vi "Get RGA Parameters.vi"(0 "Port Number":refnum<visa-resource-name>, 1 "error in (no error)":errorcluster) -> (2 "RGA Parameters":T1 {"Partial Pressure\nSensitivity Factor" format="%.3e"; "Steps/AMU" format="%.2f"; "Final Mass" format="%.2f"; "Initial Mass" format="%.2f"}, 4 "error out":errorcluster)   [LabVIEW 2025]
doc: "Author: Scott Hannahs <sth@magnet.fsu.edu>\n\nThis software is licensed for use under the “MIT License\"\nCopyright (c) 2025 Scott Hannahs, sth@sth@magnet.sthnet.net\n\nPermission is hereby granted, free of charge, to any person obtaining a copy of this software and associated documentation files (the \"Software\"), to deal in the Software without restriction, including without limitation the rights to use, copy, modify, merge, publish, distribute, sublicense, and/or sell copies of the Software, and to permit persons to whom the Software is furnished to do so, subject to the following conditions: The above copyright notice and this permission notice shall be included in all copies or substantial portions of the Software.\n\nTHE SOFTWARE IS PROVIDED \"AS IS\", WITHOUT WARRANTY OF ANY KIND, EXPRESS OR IMPLIED, INCLUDING BUT NOT LIMITED TO THE WARRANTIES OF MERCHANTABILITY, FITNESS FOR A PARTICULAR PURPOSE AND NONINFRINGEMENT. IN NO EVENT SHALL THE AUTHORS OR COPYRIGHT HOLDERS BE LIABLE FOR ANY CLAIM, DAMAGES OR OTHER LIABILITY, WHETHER IN AN ACTION OF CONTRACT, TORT OR OTHERWISE, ARISING FROM, OUT OF OR IN CONNECTION WITH THE SOFTWARE OR THE USE OR OTHER DEALINGS IN THE SOFTWARE."
uses:
  Serial Support VISA.llb/Serial Actions.ctl
panel:
  out "Serial Read":string
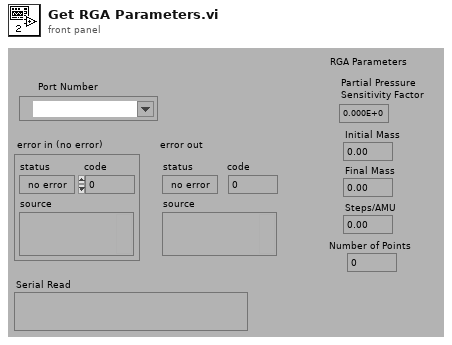
[diagram p1: front panel]
types:
  T1 = cluster{"Number of Points":u32, "Initial Mass":dbl, "Final Mass":dbl, "Steps/AMU":dbl, "Partial Pressure\nSensitivity Factor":dbl}
  T2 = typedef "Serial Actions.ctl" = enum16{"Init", "Break", "Clear Buffer", "Write", "Read", "N Bytes", "Lock", "Unlock", "Close"}
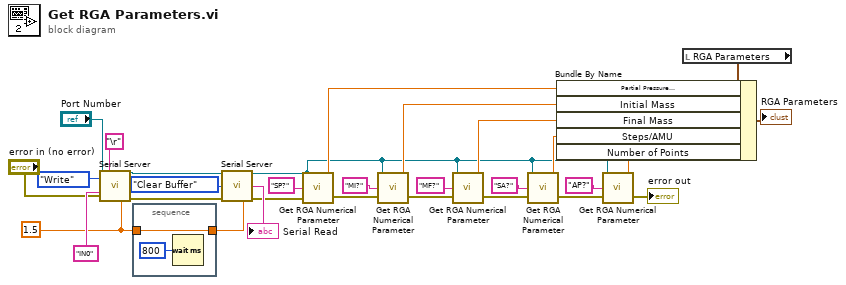
[diagram p0: block diagram]
diagram:
  w23 = 1.5
  n1 = call "Serial Server.vi"("VISA Resource Name"="Port Number", "EOT Chars (cr/lf)"="\r", "Action"=Serial_Actions."Write", "String To Send"="IN0", "error in (no error)"="error in (no error)", "Timeout Limit(sec)"=w23) -> ("dup VISA Resource Name"=w2:refnum<visa-resource-name>, "error out"=w24:errorcluster)  [unwired: 5 in, 3 out]
  n2 = stacked-sequence {
    tunnel: [w31] -> w19
    tunnel: w23 -> [w31]
    frame #0 {
      n3 = Wait (ms)(milliseconds to wait=u32 800) -> ()  [unwired: 1 out]
    }
  }
  n4 = call "Serial Server.vi"("VISA Resource Name"=w2, "Action"=Serial_Actions."Clear Buffer", "error in (no error)"=w24, "Timeout Limit(sec)"=w19) -> ("dup VISA Resource Name"=w1:refnum<visa-resource-name>, "Serial Read"=→"Serial Read":string, "error out"=w21:errorcluster)  [unwired: 7 in, 2 out]
  n5 = call "Get RGA Numerical Parameter.vi"("error in (no error)"=w21, "Command"="SP?", "Port Number"=w1) -> ("error out"=w13:errorcluster, "Parameter"=w22:dbl)  [unwired: 1 in]
  n6 = call "Get RGA Numerical Parameter.vi"("error in (no error)"=w13, "Command"="MI?" ("String To Send"), "Port Number"=w1) -> ("error out"=w15:errorcluster, "Parameter"=w10:dbl)  [unwired: 1 in]
  n7 = call "Get RGA Numerical Parameter.vi"("error in (no error)"=w15, "Command"="MF?" ("String To Send"), "Port Number"=w1) -> ("error out"=w14:errorcluster, "Parameter"=w9:dbl)  [unwired: 1 in]
  n8 = call "Get RGA Numerical Parameter.vi"("error in (no error)"=w14, "Command"="SA?" ("String To Send"), "Port Number"=w1) -> ("error out"=w12:errorcluster, "Parameter"=w8:dbl)  [unwired: 1 in]
  n9 = call "Get RGA Numerical Parameter.vi"("error in (no error)"=w12, "Command"="AP?" ("String To Send"), "Port Number"=w1) -> ("error out"=→"error out":errorcluster, "Parameter"=w7:dbl)  [unwired: 1 in]
  n10 = local read "RGA Parameters"() -> (w29:T1)
  n11 = Bundle By Name(cluster=w29, "Partial Pressure\nSensitivity Factor"=w22, "Initial Mass"=w10, "Final Mass"=w9, "Steps/AMU"=w8, "Number of Points"=w7) -> (→"RGA Parameters":T1)
